vi "Interrupt.vi"(8 "error in (no error)":errorcluster, 11 "Microscope in":refnum<class "Microscope.lvclass">) -> (0 "error out":errorcluster, 3 "Microscope out":refnum<class "Microscope.lvclass">)   [LabVIEW 2012, in "Microscope.lvclass"]
uses:
  classes/Microscope.lvclass
  typedefs/MicroscopeEvent.ctl
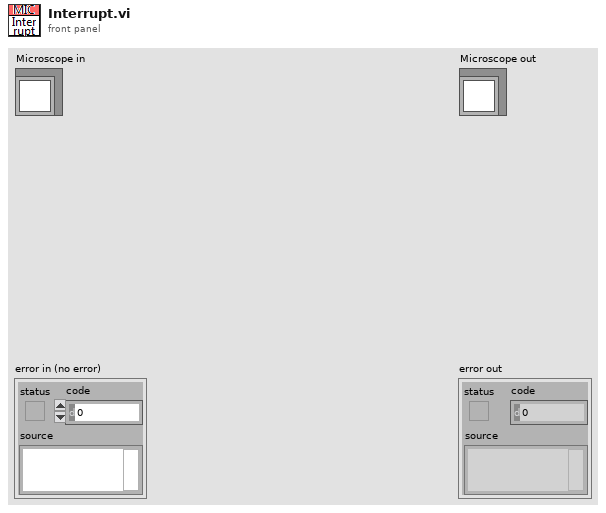
[diagram p1: front panel]
types:
  T1 = typedef "MicroscopeEvent.ctl" = enum16{"M.Wait", "M.RunRotation", "M.Flush", "M.Init", "M.InitStage", "M.InitImageData", "M.ReinitImageData", "M.ReinitImageParams", "M.GetSetParams", "M.InitFastHardware", "M.Pre-Acquire", "M.Acquire", "M.PostAcquire", "M.StopAcquire", "M.SetAcqStatusTrue", "M.SetAcqStatusFalse", "M.ClearImageData", "M.MoveStageDiscrete", "M.MoveStageToTarget1", "M.MoveStageToTarget2", "M.MoveStageToTarget3", "M.OpenShutters", "M.CloseShutters", "M.StartAcquireSequence", "M.ChangeParameters", "M.OpenStokes", "M.OpenPump", "M.RunSW"}
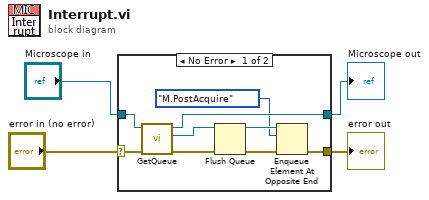
[diagram p0: block diagram]
diagram:
  n1 = case shown="No Error" "error in (no error)" {
    selector: "error in (no error)" -> [w11 w15]
    tunnel: [w6 w15] -> w3
    tunnel: [w12 w14] -> w1
    tunnel: "Microscope in" -> [w13 w14]
    frame No Error {
      n2 = call "GetQueue.vi"("error in (no error)"=w11, "Microscope in"=w13) -> ("error out"=w10:errorcluster, "Microscope events"=w9:refnum<queue>, "Microscope out"=w12:refnum<class "Microscope.lvclass">)  [unwired: 7 in]
      n3 = Flush Queue(queue=w9, error in (no error)=w10) -> (queue out=w8:refnum<queue>, error out=w5:errorcluster)  [unwired: 1 out]
      n4 = Enqueue Element At Opposite End(queue=w8, element=MicroscopeEvent."M.PostAcquire" ("Microscope events"), error in (no error)=w5) -> (error out=w6:errorcluster)  [unwired: 1 in, 2 out]
    }
    frame Error {
    }
  }
  "error out" <- w3
  "Microscope out" <- w1
